vi "Angle Distance.vi"(1 "Target Angle":dbl(knob) scale=-180.0..180.0, 2 "Current Angle":dbl(knob) scale=-180.0..180.0) -> (0 "Distance":dbl)   [LabVIEW 2019]
uses:
  <vilib>/Analysis/coordinate.llb/Angle Range (Degree).ctl
  <vilib>/Analysis/coordinate.llb/Angle Units.ctl
  <vilib>/Analysis/coordinate.llb/Wrap Angle (scalar).vi
  <vilib>/Analysis/NI_AAL_Angle.lvlib
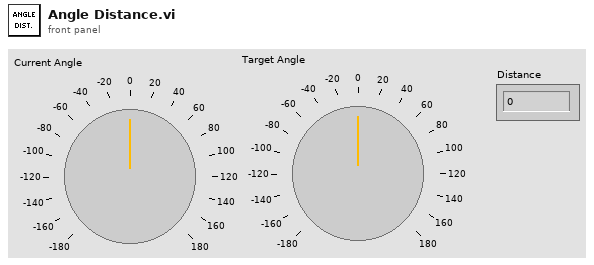
[diagram p1: front panel]
types:
  T1 = typedef "NI_AAL_Angle.lvlib/Angle Units.ctl" = i32
  T2 = typedef "NI_AAL_Angle.lvlib/Angle Range (Degree).ctl" = u16
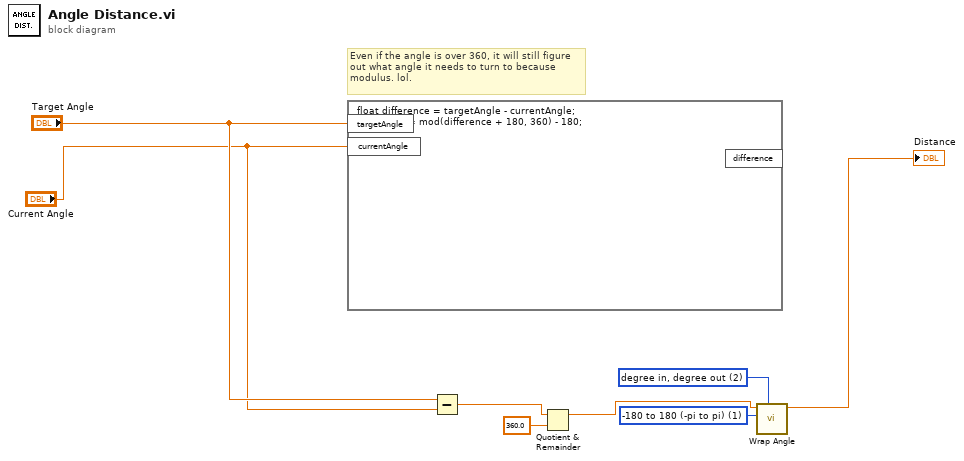
[diagram p0: block diagram]
diagram:
  w2 = T1 2 items=["radian in, radian out", "radian in, degree out", "degree in, degree out", "degree in, radian out"] ("angle units")
  w4 = T2 1 items=["none", "-180 to 180 (-pi to pi)", "0 to 360 (0 to 2pi)"] ("angle range")
  # "Even if the angle is over 360, it will still figure\nout what angle it needs to turn to because \nmodulus. lol."
  n1 = formula code="float difference = targetAngle - currentAngle;\ndifference = mod(difference + 180, 360) - 180;"("targetAngle"="Target Angle", "currentAngle"="Current Angle") -> ()  [unwired: 1 out]
  n2 = Subtract(x="Target Angle", y="Current Angle") -> (x-y=w6:dbl)
  n3 = Quotient & Remainder(x=w6, y=360.0) -> (x-y*floor(x/y)=w3:dbl)  [unwired: 1 out]
  n4 = call-poly <vilib>:"Wrap Angle.vi"("angle units"=w2, "angle range"=w4, "angle in"=w3) -> ("angle out"=→"Distance":dbl)  [unwired: 7 in, 1 out]
